vi "GetBranchName.vi"(11 "Node In":refnum<data-value>) -> (2 "Node Name Out":string, 3 "Node Out":refnum<data-value>)   [LabVIEW 2019]
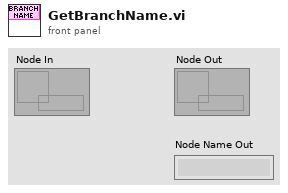
[diagram p1: front panel]
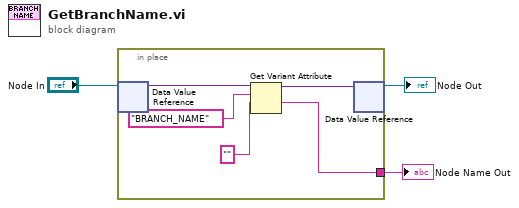
[diagram p0: block diagram]
diagram:
  n1 = in-place {
    in-place-border: [w4] -> w1
    n2 = in-place-dvr #1("Node In") -> (w8:variant)  [unwired: 1 out]
    n3 = Get Variant Attribute(Variant=w8, name="BRANCH_NAME" ("Unique Node Name"), default value (empty Variant)="") -> (duplicate Variant=w5:variant, value=w4:string)  [unwired: 1 in, 2 out]
    n4 = in-place-dvr #1(w5) -> (→"Node Out":refnum<data-value>)  [unwired: 1 out]
  }
  "Node Name Out" <- w1
